vi "helper_SCD_Setup.vi"(8 "error in":errorcluster, 11 "show ICL for debugging":bool) -> (0 "error out":errorcluster, 1 "Module Was Already Running?":bool, 2 "device open for communication?":bool, 3 "SCD out":refnum<class "SCD.lvclass">)   [LabVIEW 2020, in "horiba.test.lvlib"]
uses:
  horiba.test.lvlib
  Classes/SCD/SCD.lvclass
  Classes/DeviceManager/DeviceManager.lvlib
  <userlib>/_OpenG.lib/error/error.llb/openg_error.lvlib
panel:
  # "Connector Pane"
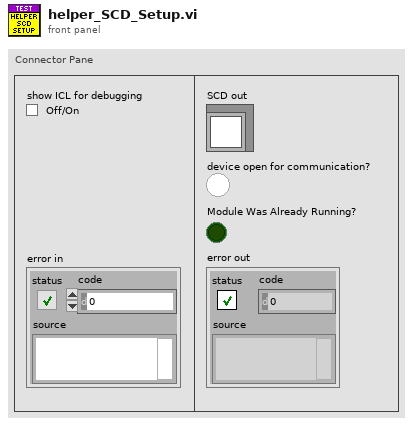
[diagram p1: front panel]
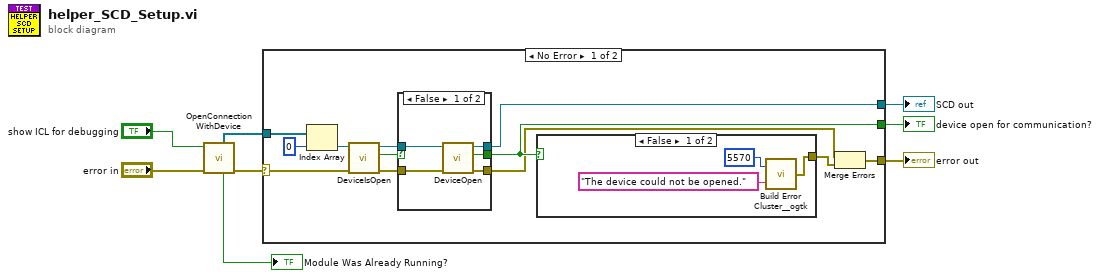
[diagram p0: block diagram]
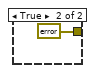
[diagram p3: hidden frame]
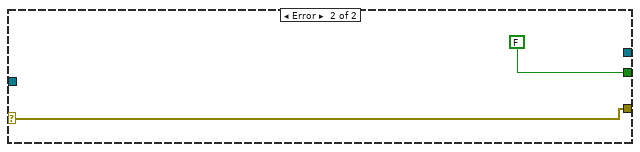
[diagram p4: hidden frame]
diagram:
  n1 = call "OpenConnectionWithDevice.vi"("error in"="error in", "show ICL for debugging"="show ICL for debugging") -> ("error out"=w5:errorcluster, "Module Was Already Running?"=→"Module Was Already Running?":bool, "SCDs"=w3:refnum<class "SCD.lvclass">[])  [unwired: 5 in, 2 out]
  n2 = case shown="No Error" w5 {
    selector: w5 -> [w12 w34]
    tunnel: w3 -> [w20 _]
    tunnel: [w18 w34] -> w7
    tunnel: [w16 FALSE ("CCD open for communication?")] -> w6
    tunnel: [w14 _] -> w2
    frame No Error {
      n3 = Index Array(array=w20, index=0) -> (element=w13:refnum<class "SCD.lvclass">)
      n4 = call-dynamic "DeviceIsOpen.vi"("error in (no error)"=w12, "SCD in"=w13) -> ("error out"=w11:errorcluster, "device is open?"=w10:bool, "SCD out"=w9:refnum<class "SCD.lvclass">)  [unwired: 6 in, 1 out]
      n5 = case shown="False" w10 {
        selector: w10 -> [_ w26]
        tunnel: [w25 w26] -> w16
        tunnel: [w24 w27] -> w15
        tunnel: [w23 w28] -> w14
        tunnel: w11 -> [w22 w27]
        tunnel: w9 -> [w21 w28]
        frame False {
          n6 = call-dynamic "DeviceOpen.vi"("error in (no error)"=w22, "SCD in"=w21) -> ("error out"=w24:errorcluster, "device is open?"=w25:bool, "SCD out"=w23:refnum<class "SCD.lvclass">)  [unwired: 6 in, 1 out]
        }
        frame True {
        }
      }
      n7 = case shown="False" w16 {
        tunnel: [w30 errorcluster {"status"=FALSE, "code"=0, "source"=""} ("error in 2")] -> w17
        frame False {
          n8 = call <userlib>:"Build Error Cluster__ogtk.vi"("String to Prepend to source (\"\")"="The device could not be opened." ("String to Prepend to source (\"\")"), "code"=5570) -> ("error out"=w30:errorcluster)
        }
        frame True {
        }
      }
      n9 = Merge Errors(w15, w17) -> (w18:errorcluster)
    }
    frame Error {
    }
  }
  "error out" <- w7
  "device open for communication?" <- w6
  "SCD out" <- w2
